vi "Remove Amplification.vi"(9 "Amplification Factor":dbl=515.0 format="%#_13g", 11 "Array":dbl[][](array[numeric])) -> (3 "Array 2":dbl[][](array[numeric]))   [LabVIEW 2018]
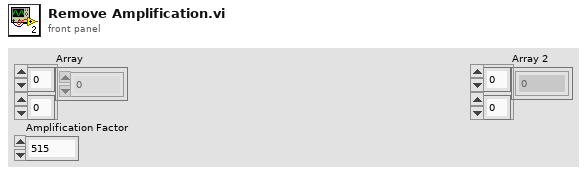
[diagram p1: front panel]
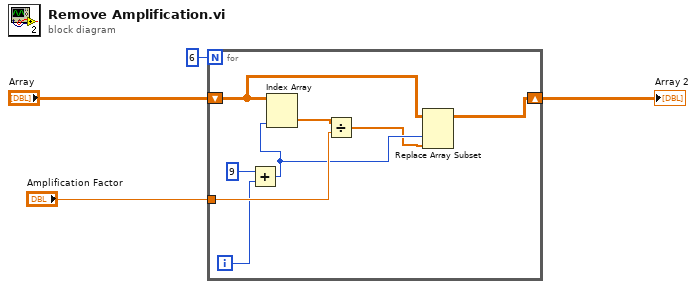
[diagram p0: block diagram]
diagram:
  n1 = for {
    N: 6 -> [_]
    tunnel: "Amplification Factor" -> [w11]
    shift-right: [w7] -> w1
    shift-left: "Array" -> [w8]
    i -> [w10]
    n2 = Add(x=9, y=w10) -> (x+y=w6:i32)
    n3 = Index Array(array=w8, index (col)=w6) -> (element=w12:dbl[])  [unwired: 1 in]
    n4 = Divide(x=w12, y=w11) -> (x/y=w5:dbl[])
    n5 = Replace Array Subset(array=w8, new element=w5, index (col)=w6) -> (w7:dbl[][])  [unwired: 1 in]
  }
  "Array 2" <- w1
